vi "Get Tau.vi"(6 "ErrorCallOn":bool, 7 "init":bool, 9 "CalType":T1=enum."LRS", 10 "Dt":dbl, 11 "X":dbl[](array[numeric])) -> (0 "B":dbl, 1 "A":dbl, 2 "e_tau":dbl, 3 "tau":dbl)   [LabVIEW 2011]
doc: "This VI uses the techniques in Everest and Atkinson [2008] to determine the decay time constant of an exponential function with no background subtraction required. There are three techniques coded with one technique (LRS) coded in both Labview and C (and compiled in a dll). According to Everest and Atkinson, the DFT routines should be on par in terms of computation time with that of the LRS while the LRS should be substantially less susceptible to noise. According to the authors, the LRS and DFT routines should proceed in about 200 us for a 1000 point data sets. A description of the techniques is given in the block diagram.\n\n1. Initialize the VI so that we only have to do certain calculations required by the routine one time. For the DFT routines, we will calculate the sine and cosine of the angular frequency (wk = 2*pi*k/(N*dt)) as well as the weights used in the DFT-5 calculation. Since the average is weighted, the average of the tau's given by each of the frequency components will be sum(w_k*tau_k)/sum(w_k) where the values are summed over 1...5. For the LRS routines, the sums over t and t^2 can be determined apriori and therefore we only need to do them when we initialize. Bundle all of these into a single cluster and pick off the values required by the different routines.\n\n2. Solve for tau using one of the routines given in Everest and Atkinson [2008]. The DFT routines are fast on both a dual core and quad core machine (on the order of 10s of microseconds) while the LRS routines both incur substantial penalties for the explicit integration (1.5 ms for the Labview based solution and 750 us for the dll based routine. The DFT-5 is less susceptible to noise than the DFT-1 while the LRS routine is significantly better at noise rejection than the DFT."
uses:
  analys_meth.ctl
  <vilib>/Analysis/baseanly.llb/Matrix Type of Inverse Matrix.ctl
  <vilib>/Analysis/7linalg.llb/Solve Linear Equations (single right hand).vi
  <vilib>/Analysis/2dsp.llb/Real FFT.vi
  <vilib>/Analysis/Matrix/Numeric/Conversions/Array To Matrix - RA2.vi
  <vilib>/Analysis/baseanly.llb/Solve Linear Equations By Cholesky.vi
  <vilib>/Analysis/NI_AALPro.lvlib
  <vilib>/Analysis/NI_AALBase.lvlib
  <vilib>/Analysis/Matrix/NI_Matrix.lvlib
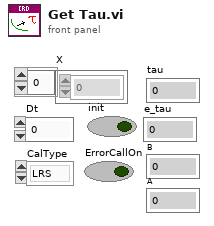
[diagram p1: front panel]
types:
  T1 = typedef "analys_meth.ctl" = enum16{"DFT-1", "DFT-5", "LRS"}
  T2 = typedef "NI_AALBase.lvlib/Matrix Type of Inverse Matrix.ctl" = enum32{"General", "Positive Definite", "Lower Triangular", "Upper Triangular"}
  T3 = typedef "NI_Matrix.lvlib/RealMatrix.ctl" = dbl[][]
  T4 = cluster{i32, dbl[], dbl[], dbl[], dbl, dbl[], dbl, dbl}
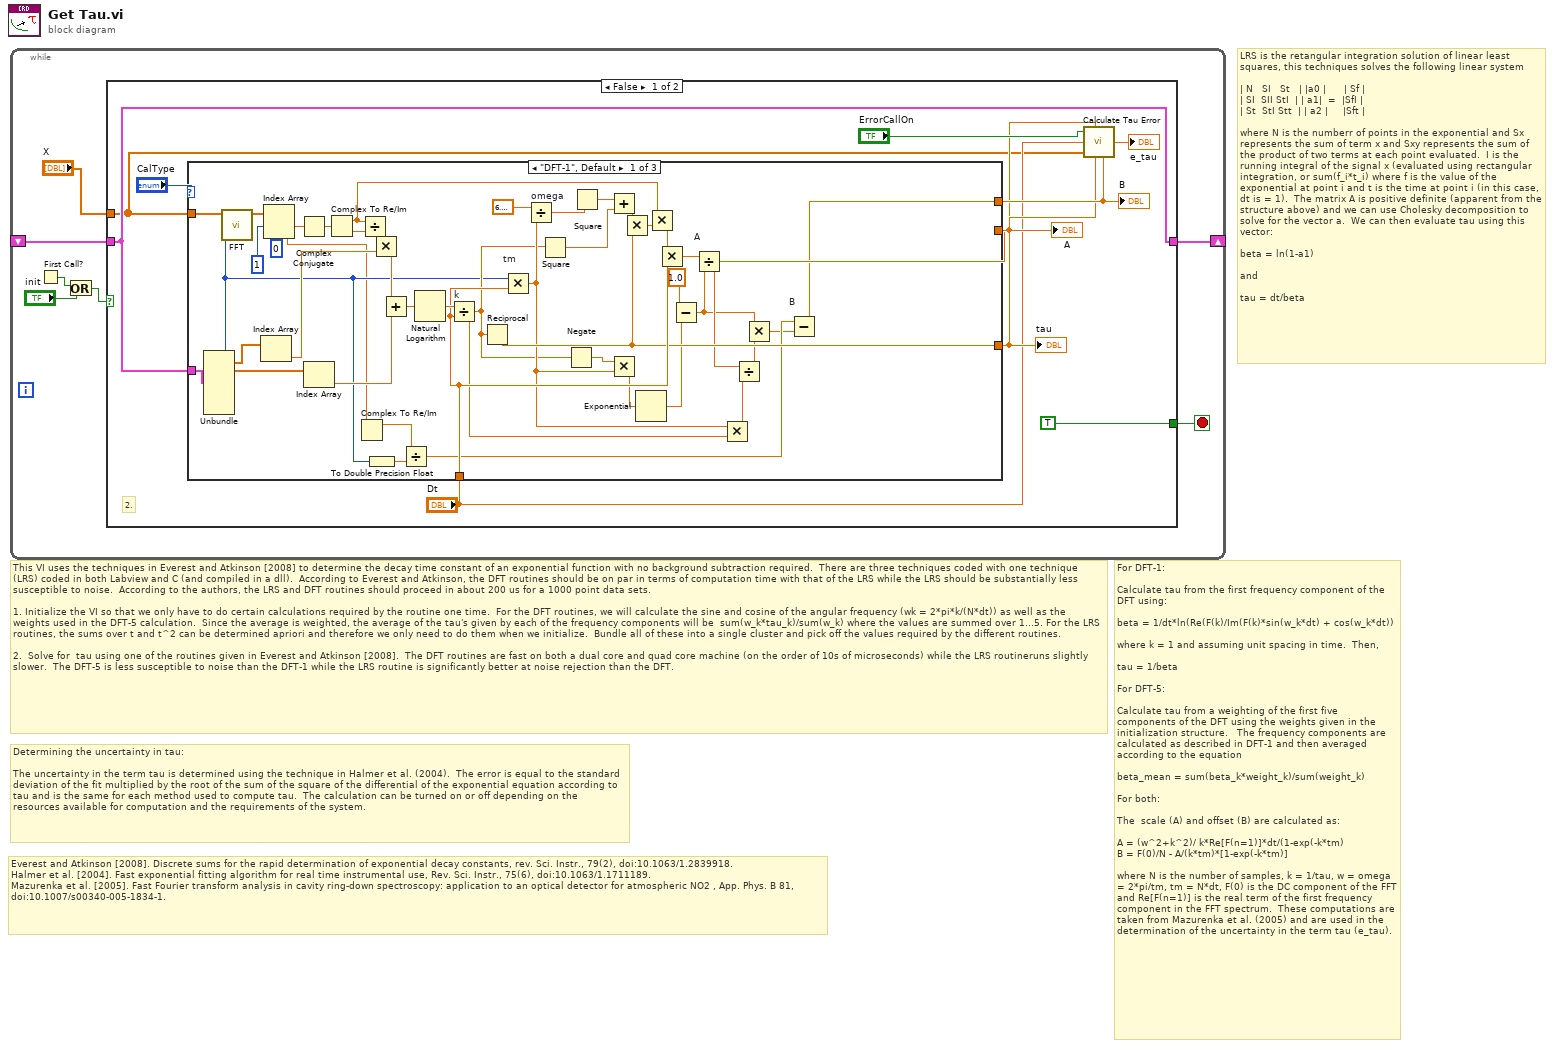
[diagram p0: block diagram]
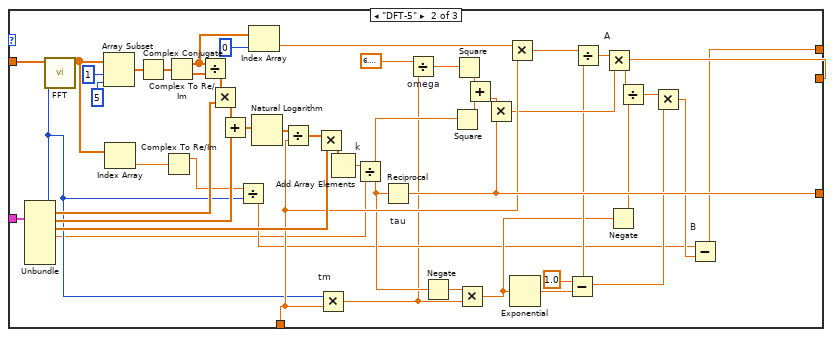
[diagram p2: hidden frame]
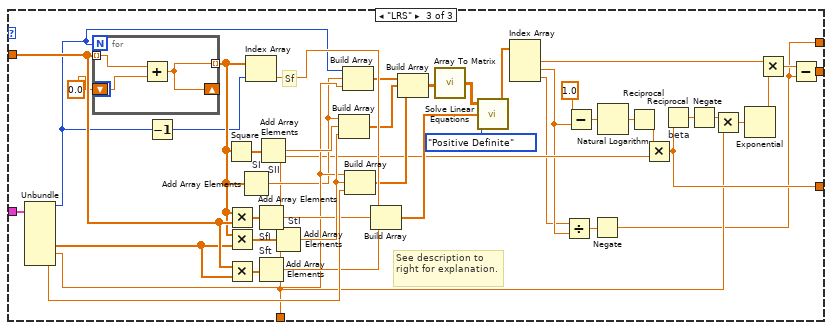
[diagram p3: hidden frame]
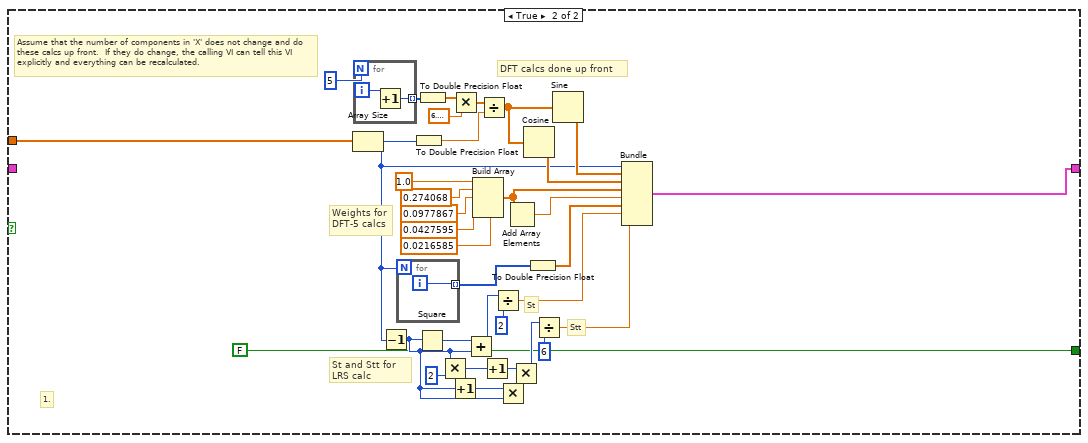
[diagram p4: hidden frame]
diagram:
  # "Determining the uncertainty in tau:\n \nThe uncertainty in the term tau is determined using the technique in Halmer et al. (2004).  The error is equal to the standard deviation of the fit multiplied by the root of the sum of the square of the differential of the exponential equation according to tau and is the same for each method used to compute tau.  The calculation can be turned on or off depending on the resources available for computation and the requirements of the system."
  # "For DFT-1:\n\nCalculate tau from the first frequency component of the DFT using:\n\nbeta = 1/dt*ln(Re(F(k)/Im(F(k)*sin(w_k*dt) + cos(w_k*dt))\n\nwhere k = 1 and assuming unit spacing in time.  Then, \n\ntau = 1/beta\n\nFor DFT-5:\n\nCalculate tau from a weighting of the first five components of the DFT using the weights given in the initialization structure.   The frequency components are calculated as described in DFT-1 and then averaged according to the equation\n\nbeta_mean = sum(beta_k*weight_k)/sum(weight_k)\n\nFor both:\n\nThe  scale (A) and offset (B) are calculated as:\n\nA = (w^2+k^2)/ k*Re[F(n=1)]*dt/(1-exp(-k*tm)\nB = F(0)/N - A/(k*tm)*[1-exp(-k*tm)]\n\nwhere N is the number of samples, k = 1/tau, w = omega = 2*pi/tm, tm = N*dt, F(0) is the DC component of the FFT and Re[F(n=1)] is the real term of the first frequency component in the FFT spectrum.  These computations are taken from Mazurenka et al. (2005) and are used in the determination of the uncertainty in the term tau (e_tau)."
  # "Everest and Atkinson [2008]. Discrete sums for the rapid determination of exponential decay constants, rev. Sci. Instr., 79(2), doi:10.1063/1.2839918.\nHalmer et al. [2004]. Fast exponential fitting algorithm for real time instrumental use, Rev. Sci. Instr., 75(6), doi:10.1063/1.1711189.\nMazurenka et al. [2005]. Fast Fourier transform analysis in cavity ring-down spectroscopy: application to an optical detector for atmospheric NO2 , App. Phys. B 81, doi:10.1007/s00340-005-1834-1."
  # "LRS is the retangular integration solution of linear least squares, this techniques solves the following linear system \n\n| N   SI   St   | |a0 |      | Sf |\n| SI  SII StI  | | a1|  =  |SfI |\n| St  StI Stt  | | a2 |     |Sft |\n\nwhere N is the numberr of points in the exponential and Sx represents the sum of term x and Sxy represents the sum of the product of two terms at each point evaluated.  I is the running integral of the signal x (evaluated using rectangular integration, or sum(f_i*t_i) where f is the value of the exponential at point i and t is the time at point i (in this case, dt is = 1).  The matrix A is positive definite (apparent from the structure above) and we can use Cholesky decomposition to solve for the vector a.  We can then evaluate tau using this vector:\n\nbeta = ln(1-a1)\n\nand \n\ntau = dt/beta"
  # "This VI uses the techniques in Everest and Atkinson [2008] to determine the decay time constant of an exponential function with no background subtraction required.  There are three techniques coded with one technique (LRS) coded in both Labview and C (and compiled in a dll).  According to Everest and Atkinson, the DFT routines should be on par in terms of computation time with that of the LRS while the LRS should be substantially less susceptible to noise.  According to the authors, the LRS and DFT routines should proceed in about 200 us for a 1000 point data sets. \n\n1. Initialize the VI so that we only have to do certain calculations required by the routine one time.  For the DFT routines, we will calculate the sine and cosine of the angular frequency (wk = 2*pi*k/(N*dt)) as well as the weights used in the DFT-5 calculation.  Since the average is weighted, the average of the tau's given by each of the frequency components will be  sum(w_k*tau_k)/sum(w_k) where the values are summed over 1...5. For the LRS routines, the sums over t and t^2 can be determined apriori and therefore we only need to do them when we initialize.  Bundle all of these into a single cluster and pick off the values required by the different routines.\n\n2.  Solve for  tau using one of the routines given in Everest and Atkinson [2008].  The DFT routines are fast on both a dual core and quad core machine (on the order of 10s of microseconds) while the LRS routineruns slightly slower.  The DFT-5 is less susceptible to noise than the DFT-1 while the LRS routine is significantly better at noise rejection than the DFT."
  n1 = while {
    shift-right: [w3] -> _
    shift-left: _ -> [w7]
    stop <- w1 stop-if-true
    n2 = First Call?() -> (First Call?: T/F=w5:bool)
    n3 = Or(x=w5, y="init") -> (x .or. y?=w6:bool)
    n4 = case shown="False" w6 {
      tunnel: "X" -> [w9 w190]
      tunnel: [w10 w183] -> w3
      tunnel: w7 -> [w10 _]
      tunnel: [TRUE FALSE] -> w1
      frame False {
        # "2."
        n5 = case shown="\"DFT-1\", Default" "CalType" {
          tunnel: w9 -> [w47 w99 w148]
          tunnel: w10 -> [w56 w98 w153]
          tunnel: "Dt" -> [w38 w88 w118]
          tunnel: [w36 w91 w121] -> w13
          tunnel: [w29 w77 w113] -> w16
          tunnel: [w24 w69 w112] -> w17
          frame "DFT-1", Default {
            n6 = Unbundle(w56) -> (w21:i32, w55:dbl[], w54:dbl[])  [unwired: 5 out]
            n7 = call-poly <vilib>:"FFT.vi"("FFT size"=w21, "X"=w47) -> ("FFT {X}"=w51:cdb[])  [unwired: 1 in, 8 out]
            n8 = Index Array(array=w55) -> (element=w53:dbl)  [unwired: 1 in]
            n9 = Index Array(array=w51, index #1=1 ("index"), index #2=0 ("index")) -> (element #1=w49:cdb, element #2=w19:cdb)
            n10 = Complex Conjugate(1:w49) -> (0:w57:cdb)
            n11 = Index Array(array=w54) -> (element=w52:dbl)  [unwired: 1 in]
            n12 = Complex To Re/Im(x + iy=w57) -> (x=w41:dbl, y=w58:dbl)
            n13 = Complex To Re/Im(x + iy=w19) -> (x=w18:dbl)  [unwired: 1 out]
            n14 = Divide(x=w41, y=w58) -> (x/y=w61:dbl)
            n15 = To Double Precision Float(number=w21) -> (double precision float=w20:dbl)
            n16 = Multiply(x=w61, y=w53) -> (x*y=w60:dbl)
            n17 = Add(x=w60, y=w52) -> (x+y=w59:dbl)
            n18 = Divide(x=w18, y=w20) -> (x/y=w30:dbl)
            n19 = Natural Logarithm(1:w59) -> (0:w48:dbl)
            n20 = Divide "k"(x=w48, y=w38) -> (x/y=w22:dbl)
            n21 = Reciprocal(x=w22) -> (1/x=w36:dbl)
            n22 = Multiply "tm"(x=w21, y=w38) -> (x*y=w23:dbl)
            n23 = Divide "omega"(x=6.283185307179586, y=w23) -> (x/y=w45:dbl)
            n24 = Square(x=w22) -> (x^2=w44:dbl)
            n25 = Negate(x=w22) -> (-x=w35:dbl)
            n26 = Square(x=w45) -> (x^2=w43:dbl)
            n27 = Add(x=w43, y=w44) -> (x+y=w42:dbl)
            n28 = Multiply(x=w35, y=w23) -> (x*y=w34:dbl)
            n29 = Multiply(x=w42, y=w36) -> (x*y=w40:dbl)
            n30 = Exponential(1:w34) -> (0:w33:dbl)
            n31 = Multiply(x=w41, y=w40) -> (x*y=w39:dbl)
            n32 = Multiply(x=w39, y=w38) -> (x*y=w32:dbl)
            n33 = Subtract(x=1.0, y=w33) -> (x-y=w27:dbl)
            n34 = Divide "A"(x=w32, y=w27) -> (x/y=w29:dbl)
            n35 = Multiply(x=w23, y=w22) -> (x*y=w28:dbl)
            n36 = Divide(x=w29, y=w28) -> (x/y=w26:dbl)
            n37 = Multiply(x=w27, y=w26) -> (x*y=w25:dbl)
            n38 = Subtract "B"(x=w30, y=w25) -> (x-y=w24:dbl)
          }
          frame "DFT-5" {
            n39 = Unbundle(w98) -> (w71:i32, w97:dbl[], w96:dbl[], w89:dbl[], w65:dbl)  [unwired: 3 out]
            n40 = call-poly <vilib>:"FFT.vi"("FFT size"=w71, "X"=w99) -> ("FFT {X}"=w74:cdb[])  [unwired: 1 in, 8 out]
            n41 = Array Subset(array=w74, index=1, length=5) -> (w104:cdb[])
            n42 = Index Array(array=w74) -> (element=w73:cdb)  [unwired: 1 in]
            n43 = Complex Conjugate(1:w104) -> (0:w102:cdb[])
            n44 = Complex To Re/Im(x + iy=w73) -> (x=w72:dbl)  [unwired: 1 out]
            n45 = Complex To Re/Im(x + iy=w102) -> (x=w64:dbl[], y=w103:dbl[])
            n46 = Divide(x=w64, y=w103) -> (x/y=w90:dbl[])
            n47 = Multiply(x=w90, y=w97) -> (x*y=w107:dbl[])
            n48 = Add(x=w107, y=w96) -> (x+y=w106:dbl[])
            n49 = Divide(x=w72, y=w71) -> (x/y=w70:dbl)
            n50 = Index Array(array=w64, index=0) -> (element=w63:dbl)
            n51 = Natural Logarithm(1:w106) -> (0:w105:dbl[])
            n52 = Divide(x=w105, y=w88) -> (x/y=w95:dbl[])
            n53 = Multiply(x=w95, y=w89) -> (x*y=w101:dbl[])
            n54 = Multiply "tm"(x=w71, y=w88) -> (x*y=w68:dbl)
            n55 = Add Array Elements(numeric array=w101) -> (sum=w100:dbl)
            n56 = Divide "k"(x=w100, y=w65) -> (x/y=w87:dbl)
            n57 = Reciprocal "tau"(x=w87) -> (1/x=w91:dbl)
            n58 = Divide "omega"(x=6.283185307179586, y=w68) -> (x/y=w66:dbl)
            n59 = Negate(x=w87) -> (-x=w86:dbl)
            n60 = Square(x=w87) -> (x^2=w94:dbl)
            n61 = Square(x=w66) -> (x^2=w93:dbl)
            n62 = Multiply(x=w86, y=w68) -> (x*y=w79:dbl)
            n63 = Add(x=w93, y=w94) -> (x+y=w92:dbl)
            n64 = Multiply(x=w92, y=w91) -> (x*y=w82:dbl)
            n65 = Multiply(x=w63, y=w88) -> (x*y=w83:dbl)
            n66 = Exponential(1:w79) -> (0:w85:dbl)
            n67 = Subtract(x=1.0, y=w85) -> (x-y=w80:dbl)
            n68 = Divide(x=w83, y=w80) -> (x/y=w81:dbl)
            n69 = Multiply "A"(x=w81, y=w82) -> (x*y=w77:dbl)
            n70 = Negate(x=w79) -> (-x=w78:dbl)
            n71 = Divide(x=w77, y=w78) -> (x/y=w76:dbl)
            n72 = Multiply(x=w76, y=w80) -> (x*y=w75:dbl)
            n73 = Subtract "B"(x=w70, y=w75) -> (x-y=w69:dbl)
          }
          frame "LRS" {
            # "See description to right for explanation."
            # "Sf"
            n74 = Unbundle(w153) -> (w128:i32, w147:dbl[], w127:dbl, w144:dbl)  [unwired: 4 out]
            n75 = for {
              N: w128 -> [_]
              tunnel: w148 -> [w156] mode=indexing
              tunnel: [w154] -> w130 mode=indexing
              shift-right: [w154] -> _
              shift-left: 0.0 -> [w155]
              n76 = Add(x=w156, y=w155) -> (x+y=w154:dbl)
            }
            n77 = Decrement(x=w128) -> (x-1=w129:i32)
            n78 = Square(x=w130) -> (x^2=w151:dbl[])
            n79 = Multiply(x=w130, y=w148) -> (x*y=w150:dbl[])
            n80 = Multiply(x=w130, y=w147) -> (x*y=w149:dbl[])
            n81 = Multiply(x=w148, y=w147) -> (x*y=w141:dbl[])
            n82 = Add Array Elements "SI"(numeric array=w130) -> (sum=w126:dbl)
            n83 = Index Array(array=w130, index=w129) -> (element=w143:dbl)
            n84 = Add Array Elements "SfI"(numeric array=w150) -> (sum=w142:dbl)
            n85 = Add Array Elements "Sft"(numeric array=w141) -> (sum=w140:dbl)
            n86 = Add Array Elements "SII"(numeric array=w151) -> (sum=w146:dbl)
            n87 = Add Array Elements "StI"(numeric array=w149) -> (sum=w145:dbl)
            n88 = Build Array(w126, w146, w145) -> (w137:dbl[])
            n89 = Build Array(w128, w126, w127) -> (w138:dbl[])
            n90 = Build Array(w127, w145, w144) -> (w136:dbl[])
            n91 = Build Array(w143, w142, w140) -> (w139:dbl[])
            n92 = Build Array(w138, w137, w136) -> (w135:dbl[][])
            n93 = call-poly <vilib>:"Array To Matrix.vi"("Real 2D Array"=w135) -> ("Real Matrix"=w134:T3)
            n94 = call-poly <vilib>:"Solve Linear Equations.vi"("matrix type"=Matrix_Type_of_Inverse_Matrix."Positive Definite", "Known Vector"=w139, "Input Matrix"=w134) -> ("Solution Vector"=w123:dbl[])  [unwired: 1 out]
            n95 = Index Array(array=w123) -> (element #1=w110:dbl, element #2=w115:dbl, element #3=w114:dbl)  [unwired: 3 in]
            n96 = Divide(x=w114, y=w115) -> (x/y=w122:dbl)
            n97 = Subtract(x=1.0, y=w115) -> (x-y=w132:dbl)
            n98 = Negate(x=w122) -> (-x=w112:dbl)
            n99 = Natural Logarithm(1:w132) -> (0:w131:dbl)
            n100 = Reciprocal(x=w131) -> (1/x=w125:dbl)
            n101 = Multiply(x=w125, y=w118) -> (x*y=w121:dbl)
            n102 = Reciprocal "beta"(x=w121) -> (1/x=w120:dbl)
            n103 = Negate(x=w120) -> (-x=w119:dbl)
            n104 = Multiply(x=w119, y=w118) -> (x*y=w117:dbl)
            n105 = Exponential(1:w117) -> (0:w111:dbl)
            n106 = Multiply(x=w110, y=w111) -> (x*y=w116:dbl)
            n107 = Subtract(x=w116, y=w112) -> (x-y=w113:dbl)
          }
        }
        "tau" <- w13
        "A" <- w16
        "B" <- w17
        n108 = call "Calculate Tau Error.vi"("CalErr?"="ErrorCallOn", "tau"=w13, "Dt"="Dt", "X"=w9, "A"=w16, "B"=w17) -> ("e_tau"=→"e_tau":dbl)  [unwired: 3 in]
      }
      frame True {
        # "1."
        # "Assume that the number of components in 'X' does not change and do these calcs up front.  If they do change, the calling VI can tell this VI explicitly and everything can be recalculated."
        # "DFT calcs done up front"
        # "St and Stt for LRS calc"
        # "Weights for DFT-5 calcs"
        # "Stt"
        # "St"
        n109 = Array Size(array=w190) -> (size(s)=w160:i32)
        n110 = for {
          N: 5 -> [_]
          tunnel: [w193] -> w186 mode=indexing
          i -> [w194]
          n111 = Increment(x=w194) -> (x+1=w193:i32)
        }
        n112 = Decrement(x=w160) -> (x-1=w161:i32)
        n113 = for {
          N: w160 -> [_]
          tunnel: [w192] -> w163 mode=indexing
          i -> [w192]
        }
        n114 = To Double Precision Float(number=w160) -> (double precision float=w174:dbl)
        n115 = Square(x=w161) -> (x^2=w173:i32)
        n116 = To Double Precision Float(number=w186) -> (double precision float=w187:dbl[])
        n117 = Multiply(x=w161, y=2) -> (x*y=w169:i32)
        n118 = Increment(x=w161) -> (x+1=w168:i32)
        n119 = Multiply(x=w187, y=6.283185307179586) -> (x*y=w188:dbl[])
        n120 = Add(x=w173, y=w161) -> (x+y=w172:i32)
        n121 = Build Array(1.0, 0.274068, 0.0977867, 0.0427595, 0.0216585) -> (w177:dbl[])
        n122 = Divide(x=w188, y=w174) -> (x/y=w189:dbl[])
        n123 = Increment(x=w169) -> (x+1=w166:i32)
        n124 = Divide(x=w172, y=2) -> (x/y=w159:dbl)
        n125 = Multiply(x=w168, y=w161) -> (x*y=w167:i32)
        n126 = Add Array Elements(numeric array=w177) -> (sum=w176:dbl)
        n127 = Multiply(x=w166, y=w167) -> (x*y=w165:i32)
        n128 = Cosine(x=w189) -> (cos(x)=w184:dbl[])
        n129 = To Double Precision Float(number=w163) -> (double precision float=w162:dbl[])
        n130 = Divide(x=w165, y=6) -> (x/y=w158:dbl)
        n131 = Sine(x=w189) -> (sin(x)=w185:dbl[])
        n132 = Bundle(w160, w185, w184, w177, w176, w162, w159, w158) -> (w183:T4)  [unwired: 1 out]
      }
    }
  }
